vi "Initializer.vi"(8 "error in (no error)":errorcluster, 11 "UDP_Sender in":refnum<class "UDP_Sender.lvclass">) -> (0 "error out":errorcluster, 3 "UDP_Sender out":refnum<class "UDP_Sender.lvclass">)   [LabVIEW 2021, in "UDP_Sender.lvclass"]
uses:
  UDP_Sender.lvclass
  UDP_Comm/UDP_Comm.lvclass
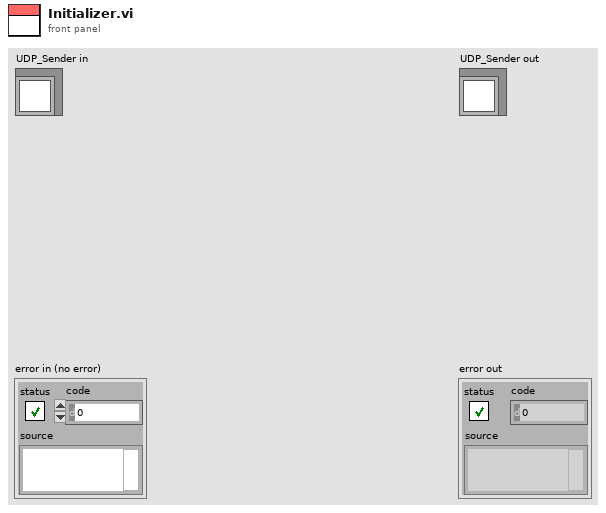
[diagram p1: front panel]
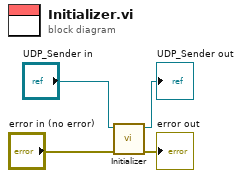
[diagram p0: block diagram]
diagram:
  n1 = call-parent "Initializer.vi"("error in (no error)"="error in (no error)", "UDP_Comm in"="UDP_Sender in") -> ("error out"=→"error out":errorcluster, "UDP_Comm out"=→"UDP_Sender out":refnum<class "UDP_Sender.lvclass">)  [unwired: 8 in]
